vi "AWS-S3-ProgressCallbackDownload.vi"(4 "Initial Data":T1, 5 "Event Data":cluster{"sender":refnum<k24>, "e":refnum<k24>}, 6 "Control Ref":refnum<k24>, 7 "Event Common Data":T2) -> ()   [LabVIEW 2012, in "AWS-S3-API.lvclass"]
uses:
  AWS-S3-API.lvclass
  C:/Users/Jack/repo/aws/AWS-SDK/AWSSDK.dll
  repo/aws/AWS-SDK/AWSSDK.dll
  AWS-S3-Transfer-Progress.ctl
  AWS-S3-Transfer-Header.ctl
panel:
  # "Inputs"
  # "Outputs"
  # "No Outputs - this VI\nis fire and forget"
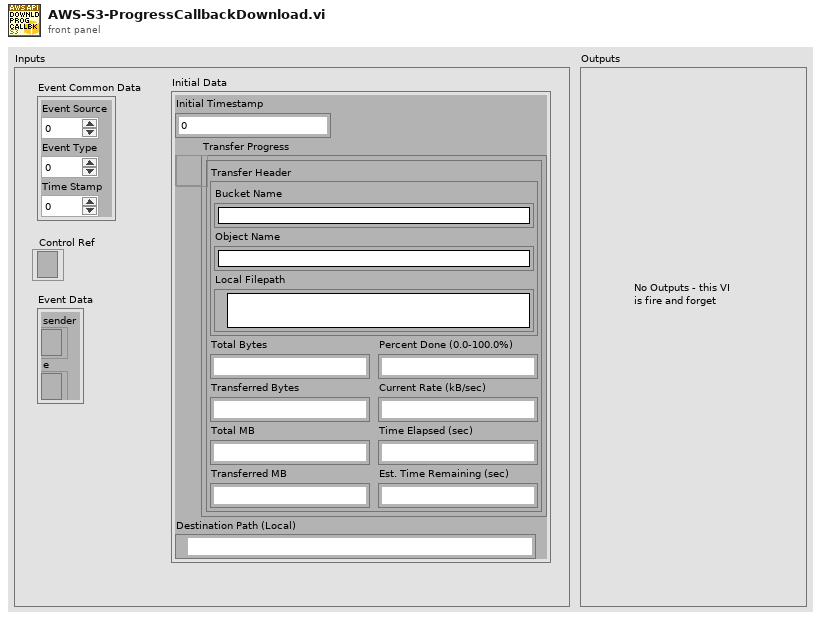
[diagram p1: front panel]
types:
  T1 = cluster{"Initial Timestamp":u32, "Transfer Progress":refnum<user-event>, "Destination Path (Local)":path}
  T2 = cluster{"Event Source":i32, "Event Type":u32, "Time Stamp":u32}
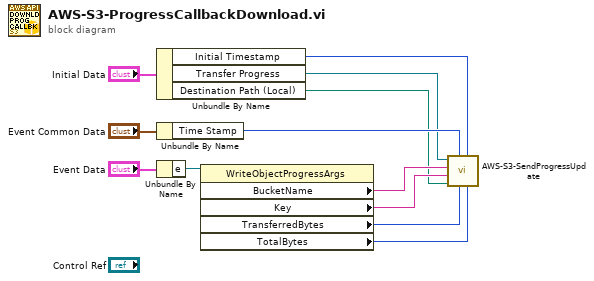
[diagram p0: block diagram]
diagram:
  n1 = Unbundle By Name("Initial Data") -> ("Initial Timestamp"=w1:u32, "Transfer Progress"=w2:refnum<user-event>, "Destination Path (Local)"=w3:path)
  n2 = Unbundle By Name("Event Common Data") -> ("Time Stamp"=w8:u32)
  n3 = Unbundle By Name("Event Data") -> ("e"=w9:refnum<k24>)
  n4 = property class="WriteObjectProgressArgs"(reference=w9) -> ("BucketName"=w7:string, "Key"=w6:string, "TransferredBytes"=w5:i64, "TotalBytes"=w4:i64)  [unwired: 1 in, 2 out]
  n5 = call "AWS-S3-SendProgressUpdate.vi"("TotalBytes"=w4, "Initial Timestamp"=w1, "TransferredBytes"=w5, "Time Stamp"=w8, "Local Filepath"=w3, "Key"=w6, "BucketName"=w7, "User Event in"=w2) -> ()  [unwired: 4 in]
